vi "get_operation_ID_from_DB.vi"(6 "results_from_PLC":u8[](array[numeric]), 7 "SQL_connection_reference":T3, 8 "error_in":errorcluster, 9 "station":T1, 11 "station_number":u16) -> (0 "error_out":errorcluster, 2 "operation_status":T2, 3 "operation_ID":string, 4 "part_ID":string)   [LabVIEW 2020]
uses:
  <vilib>/addons/database/Connection.llb/Conn ObjectReference.ctl
  SQL_statuses.ctl
  station.ctl
  FGV/SQL_part_ID_buffer/FGV_SQL_part_ID_buffer.ctl
  _misc/byte_array_parser/to_string.vi
  <vilib>/addons/database/_DB Variant To Data/Database Variant To Data.xnode
  <vilib>/addons/database/NI_Database_API.lvlib
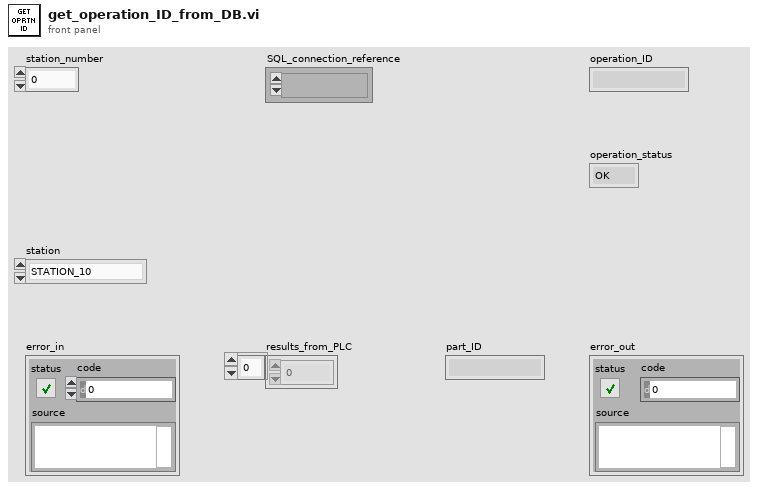
[diagram p1: front panel]
types:
  T1 = typedef "station.ctl" = enum16{"STATION_10", "STATION_20", "STATION_30", "STATION_40", "STATION_50", "STATION_60", "STATION_70", "STATION_80", "STATION_90", "STATION_100", "STATION_110", "STATION_120", "STATION_165", "MAIN"}
  T2 = typedef "SQL_statuses.ctl" = enum16{"OK", "PART_IN_OPERATION", "PART_DOES_NOT_EXIST", "OPERATION_DOES_NOT_EXIST", "OPERATOR_DOES_NOT_EXIST", "PART_NOT_IN_OPERATION"}
  T3 = typedef "NI_Database_API.lvlib/Conn ObjectReference.ctl" = refnum<k1>
  T4 = typedef "FGV_SQL_part_ID_buffer.ctl" = enum16{"initialize", "buffer_serial_ID", "get_ID_for_name"}
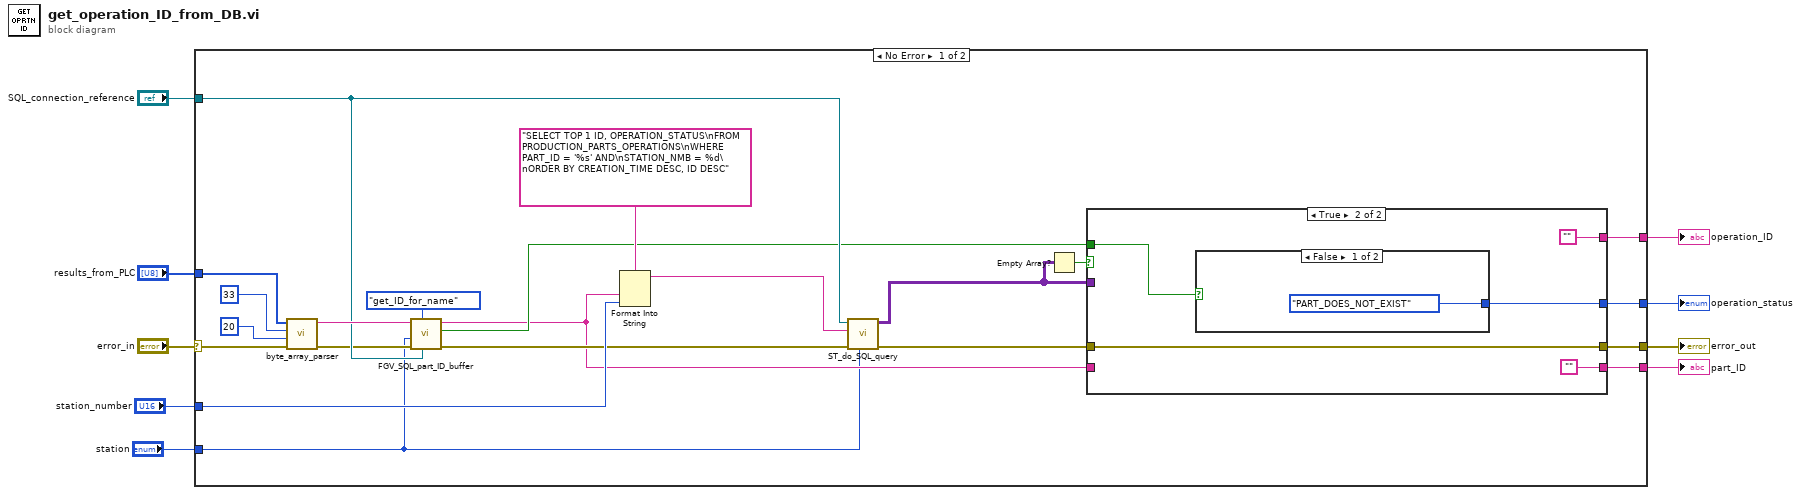
[diagram p0: block diagram]
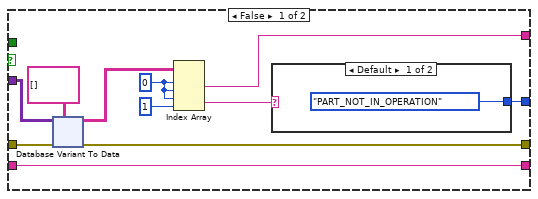
[diagram p2: hidden frame]
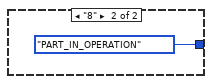
[diagram p3: hidden frame]
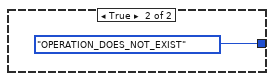
[diagram p4: hidden frame]
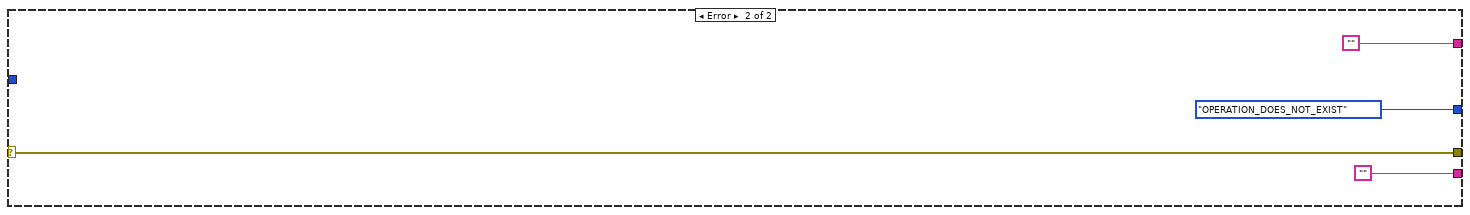
[diagram p5: hidden frame]
diagram:
  n1 = case shown="No Error" "error_in" {
    selector: "error_in" -> [w30 w99]
    tunnel: "SQL_connection_reference" -> [w24 _]
    tunnel: [w21 w99] -> w8
    tunnel: "results_from_PLC" -> [w31 _]
    tunnel: [w23 ""] -> w5
    tunnel: "station_number" -> [w22 _]
    tunnel: [w20 SQL_statuses."OPERATION_DOES_NOT_EXIST" ("SQL_statuses")] -> w3
    tunnel: [w18 ""] -> w2
    tunnel: "station" -> [w10 _]
    frame No Error {
      n2 = call-poly "byte_array_parser.vi"("error_in"=w30, "string_length"=20, "variable_start_index"=33, "byte_array"=w31) -> ("error_out"=w19:errorcluster, "string"=w25:string)  [unwired: 6 in]
      n3 = call "FGV_SQL_part_ID_buffer.vi"("connection reference"=w24, "options"=FGV_SQL_part_ID_buffer."get_ID_for_name", "error_in"=w19, "station"=w10, "PART_SERIAL"=w25) -> ("error_out"=w14:errorcluster, "Part exists?"=w12:bool, "ID_out"=w11:string)  [unwired: 4 in]
      n4 = Format Into String(format string="SELECT TOP 1 ID, OPERATION_STATUS\nFROM PRODUCTION_PARTS_OPERATIONS\nWHERE PART_ID = '%s' AND\nSTATION_NMB = %d\nORDER BY CREATION_TIME DESC, ID DESC", w11, w22) -> (resulting string=w17:string)  [unwired: 2 in, 1 out]
      n5 = call "ST_do_SQL_query.vi"("station"=w10, "error_in"=w14, "SQL_query"=w17, "SQL_connection_reference"=w24) -> ("error_out"=w13:errorcluster, "recordset_out"=w15:variant[][])  [unwired: 6 in]
      n6 = Empty Array?(array=w15) -> (empty?=w16:bool)
      n7 = case shown="True" w16 {
        tunnel: w15 -> [w42 _]
        tunnel: [w35 ""] -> w23
        tunnel: w13 -> [w40 w92]
        tunnel: [w39 w92] -> w21
        tunnel: [w33 w90] -> w20
        tunnel: w12 -> [_ w91]
        tunnel: [w32 ""] -> w18
        tunnel: w11 -> [w32 _]
        frame False {
          w37 = 0 ("index (row)")
          n8 = xnode "Database Variant To Data"("database variant"=w42, "error in (no error)"=w40, "type"=string[][] []) -> ("data"=w38:string[][], "error out"=w39:errorcluster)
          n9 = Index Array(array=w38, index (row) #1=w37, index (col) #1=w37, index (row) #2=w37, index (col) #2=1 ("disabled index (col)")) -> (element #1=w35:string, element #2=w34:string)
          n10 = case shown="Default" w34 {
            tunnel: [SQL_statuses."PART_NOT_IN_OPERATION" ("SQL_statuses") SQL_statuses."PART_IN_OPERATION" ("SQL_statuses")] -> w33
            frame Default {
            }
            frame "8" {
            }
          }
        }
        frame True {
          n11 = case shown="False" w91 {
            tunnel: [SQL_statuses."PART_DOES_NOT_EXIST" ("operation_status") SQL_statuses."OPERATION_DOES_NOT_EXIST" ("operation_status")] -> w90
            frame False {
            }
            frame True {
            }
          }
        }
      }
    }
    frame Error {
    }
  }
  "error_out" <- w8
  "operation_ID" <- w5
  "operation_status" <- w3
  "part_ID" <- w2
